vi "Read SHV Syringe Vacuum Gauge.vi"(8 "error in (no error)":errorcluster, 11 "Stepper in":refnum<class "Stepper.lvclass">) -> (0 "error out":errorcluster, 2 "Data":dbl, 3 "Stepper out":refnum<class "Stepper.lvclass">)   [LabVIEW 2015, in "Stepper.lvclass"]
uses:
  Stepper.lvclass
  Stepper.lvclass/Stepper.ctl
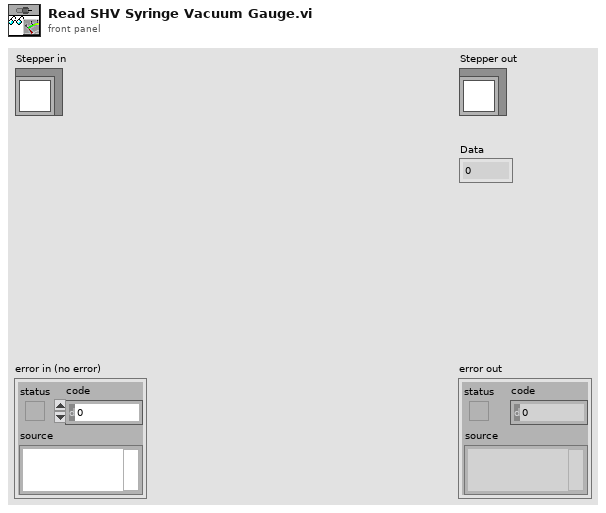
[diagram p1: front panel]
types:
  T1 = typedef "Vacuum State Cluster.ctl" = cluster{"Vacuum State":T2, "Pressure":dbl, "Raw Pressure":dbl, "d/dt":dbl}
  T2 = typedef "Vacuum State Enumerator.ctl" = enum16{"Pressure Rising", "Plateau", "Pressure Dropping", "Valley", "Low Valley", "Leak", "Unknown"}
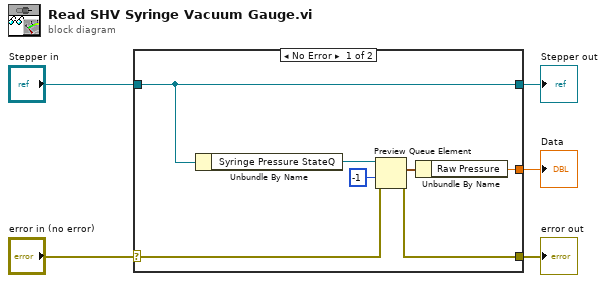
[diagram p0: block diagram]
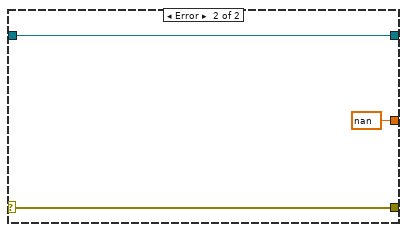
[diagram p2: hidden frame]
diagram:
  n1 = case shown="No Error" "error in (no error)" {
    selector: "error in (no error)" -> [w10 w14]
    tunnel: [w9 w14] -> w4
    tunnel: [w12 w15] -> w2
    tunnel: "Stepper in" -> [w12 w15]
    tunnel: [w6 nan] -> w1
    frame No Error {
      n2 = Unbundle By Name(w12) -> ("Syringe Pressure StateQ"=w11:refnum<queue>)
      n3 = Preview Queue Element(queue=w11, timeout in ms (-1)=-1, error in (no error)=w10) -> (element=w8:T1, error out=w9:errorcluster)  [unwired: 2 out]
      n4 = Unbundle By Name(w8) -> ("Raw Pressure"=w6:dbl)
    }
    frame Error {
    }
  }
  "error out" <- w4
  "Stepper out" <- w2
  "Data" <- w1
